vi "eat.vi"(8 "error in (no error)":errorcluster, 11 "Dog in":refnum<class "Dog.lvclass">) -> (0 "error out":errorcluster, 3 "Dog out":refnum<class "Dog.lvclass">)   [LabVIEW 2021, in "Dog.lvclass"]
uses:
  Dog.lvclass
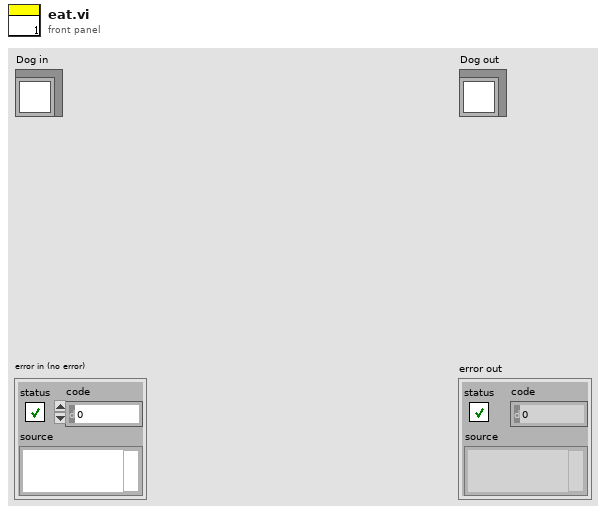
[diagram p1: front panel]
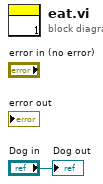
[diagram p0: block diagram]
diagram:
  "Dog out" <- "Dog in"
